vi "FunctDataMgr.Test Start.vi"(4 "Reset Data":bool=TRUE, 6 "StartTime":timestamp, 7 "Mode":string, 8 "error in (no error)":errorcluster, 9 "SN":string, 10 "Sequence":string, 11 "FunctDataMgr in":refnum<class "FunctDataMgr.lvclass">) -> (0 "error out":errorcluster, 3 "FunctDataMgr out":refnum<class "FunctDataMgr.lvclass">)   [LabVIEW 2018, in "FunctDataMgr.lvclass"]
uses:
  FunctDataMgr.lvclass
  FunctDataMgr.lvclass/FunctDataMgr.ctl
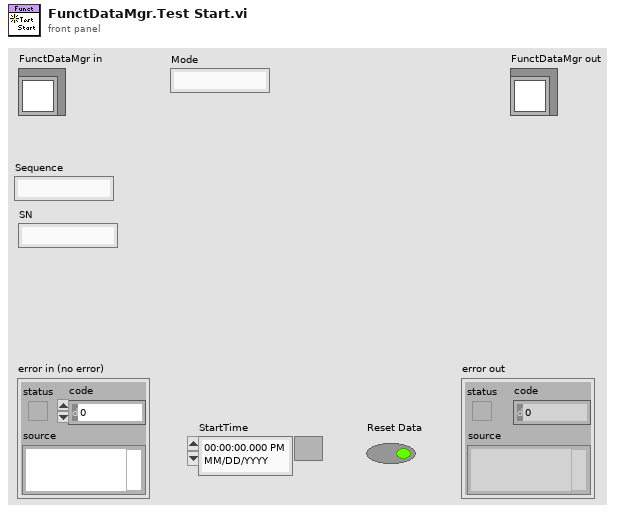
[diagram p1: front panel]
types:
  T1 = cluster{"Sequence":string, "Mode":string, "SN":string, "StartTime":timestamp, "Pos":i32}
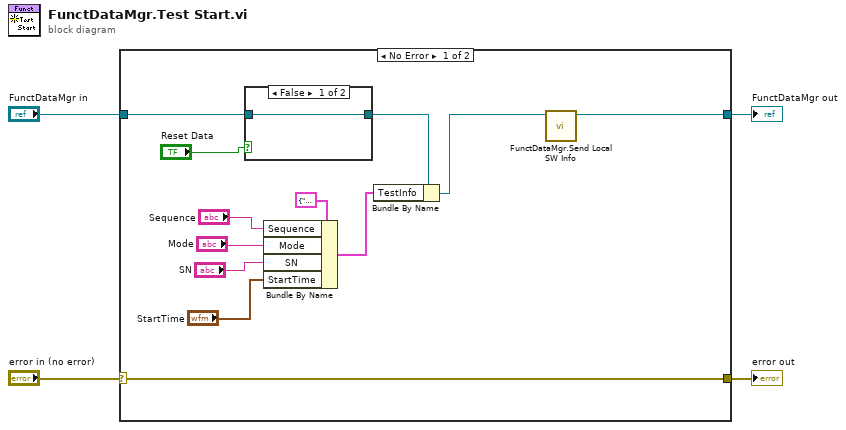
[diagram p0: block diagram]
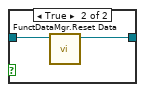
[diagram p2: hidden frame]
diagram:
  n1 = case shown="No Error" "error in (no error)" {
    selector: "error in (no error)" -> [w16 w21]
    tunnel: [w16 w21] -> w3
    tunnel: [w6 w20] -> w1
    tunnel: "FunctDataMgr in" -> [w9 w20]
    frame No Error {
      n2 = case shown="False" "Reset Data" {
        tunnel: w9 -> [w17 w19]
        tunnel: [w17 w18] -> w8
        frame False {
        }
        frame True {
          n3 = call "FunctDataMgr.Reset Data.vi"("FunctDataMgr in"=w19) -> ("FunctDataMgr out"=w18:refnum<class "FunctDataMgr.lvclass">)  [unwired: 9 in, 1 out]
        }
      }
      n4 = Bundle By Name(cluster=T1 {"Sequence"="", "Mode"="", "SN"="", "StartTime"=timestamp(0 s since 1904-01-01), "Pos"=0} ("TestInfo"), "Sequence"="Sequence", "Mode"="Mode", "SN"="SN", "StartTime"="StartTime") -> (w14:T1)
      n5 = Bundle By Name(cluster=w8, "TestInfo"=w14) -> (w7:refnum<class "FunctDataMgr.lvclass">)
      n6 = call "FunctDataMgr.Send Local SW Info.vi"("FunctDataMgr in"=w7) -> ("FunctDataMgr out"=w6:refnum<class "FunctDataMgr.lvclass">)  [unwired: 9 in, 1 out]
    }
    frame Error {
    }
  }
  "error out" <- w3
  "FunctDataMgr out" <- w1
